vi "Autonomous Independent.vi"   [LabVIEW 2012]
doc: "This VI is called when autonomous begins, and will automatically be terminated when autonomous ends. You can carry out timed or sensor driven robot movement independently without needing to return to the caller."
uses:
  <vilib>/Rock Robotics/WPI/CAN/Jaguar/SubVIs/WPI_CANJaguar_ControlMode.ctl
  <vilib>/Rock Robotics/WPI/CAN/Jaguar/SubVIs/WPI_CANJaguar_PositionReference.ctl
  <vilib>/Rock Robotics/WPI/CAN/Jaguar/SubVIs/WPI_CANJaguar_SpeedReference.ctl
  Robot Global Data.vi
  <vilib>/Rock Robotics/WPI/Solenoid/Deprecated/WPI_SolenoidSetBool.vi
  <vilib>/Rock Robotics/WPI/Joystick/WPI_JoystickGetSetRefNum.vi
types:
  T1 = typedef "WPI_JoystickDevRef.ctl" = cluster{"Device":T2}
  T2 = typedef "WPI_JoystickDeviceEnum.ctl" = enum16{"USB 1", "USB 2", "USB 3", "USB 4", "Kinect 1", "Kinect 2"}
  T3 = cluster{"axis 1 (x)":dbl, "axis 2 (y)":dbl, "axis 3 (throttle)":dbl, "axis 4":dbl, "axis 5":dbl, "axis 6":dbl}
  T4 = typedef "WPI_MotorControlDeviceRef.ctl" = cluster{"DeviceStatus":errorcluster, "Type":enum16{"PWM", "CAN"}, "PWM":cluster{"Digital Module":T5, "PWM Channel":T6, "DeadBand":T7}, "CAN":cluster{"Device Number":u8, "Control Mode":T8, "Semaphore":T9, "Max Vout":dbl}, "Invert":bool, "TransformRef":T10, "InvTransformRef":T10}
  T5 = typedef "FPGA_TypedefDigitalModule.ctl" = enum16{"Digital Module 1", "Digital Module 2"}
  T6 = typedef "FPGA_DIOPWMChannel.ctl" = enum8{"PWM 1", "PWM 2", "PWM 3", "PWM 4", "PWM 5", "PWM 6", "PWM 7", "PWM 8", "PWM 9", "PWM 10", "Invalid"}
  T7 = typedef "WPI_PWMDeadband.ctl" = cluster{"Name":string, "maxPositivePwm":i32, "minPositivePwm":i32, "centerPwm":i32, "maxNegativePwm":i32, "minNegativePwm":i32, "angularRange":u16}
  T8 = typedef "WPI_CANJaguar_ControlMode.ctl" = enum8{"Percent VBus", "Current", "Speed", "Position", "Voltage"}
  T9 = typedef "Semaphore RefNum" = refnum<k1>
  T10 = typedef "WPI_PWMTransform_ConPane.ctl" = refnum<vi>
  T11 = typedef "WPI_SolenoidDevRef.ctl" = cluster{"DevStatus":errorcluster, "Solenoid Module":T12, "Forward Solenoid Channel":T13, "Reverse Solenoid Channel":T13}
  T12 = typedef "FPGA_TypedefSolenoidModule.ctl" = enum16{"Solenoid Module 1", "Solenoid Module 2"}
  T13 = typedef "WPI_SolenoidChannel.ctl" = enum8{"Solenoid 1", "Solenoid 2", "Solenoid 3", "Solenoid 4", "Solenoid 5", "Solenoid 6", "Solenoid 7", "Solenoid 8", "Invalid"}
  T14 = typedef "WPI_CANJaguar_PositionReference.ctl" = u8
  T15 = typedef "WPI_CANJaguar_SpeedReference.ctl" = u8
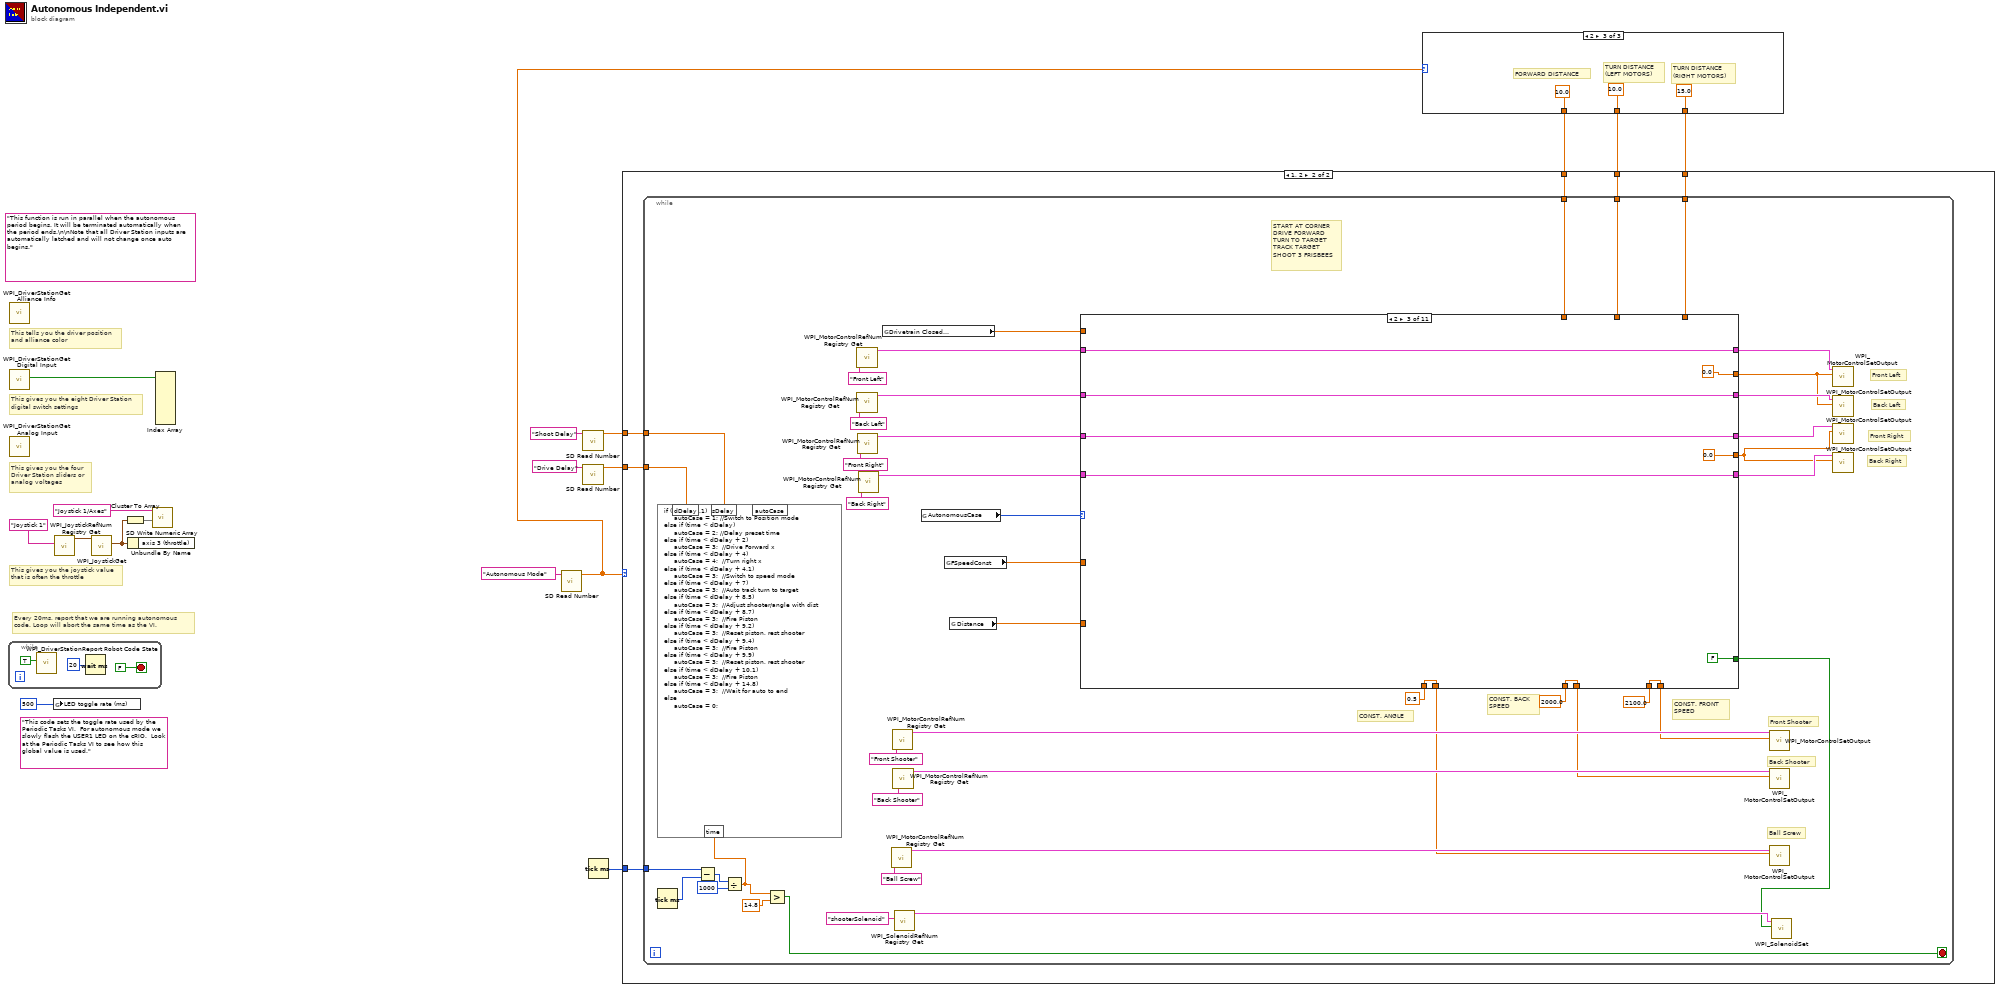
[diagram p0: block diagram]
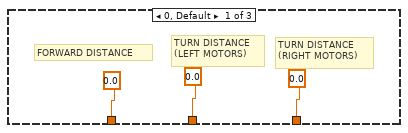
[diagram p2: hidden frame]
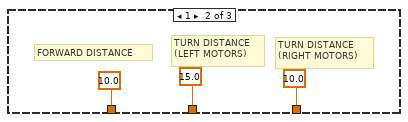
[diagram p3: hidden frame]
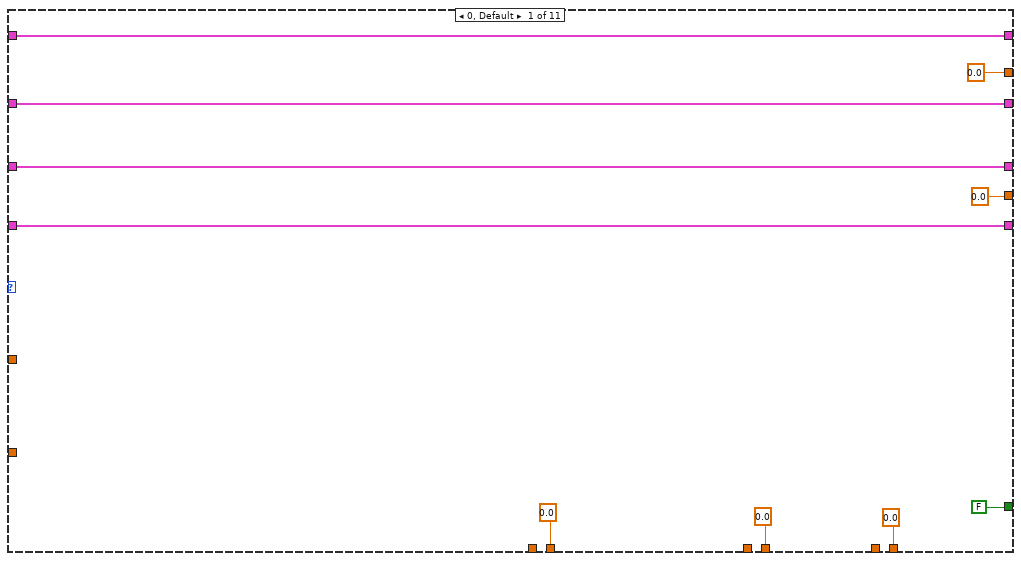
[diagram p5: hidden frame]
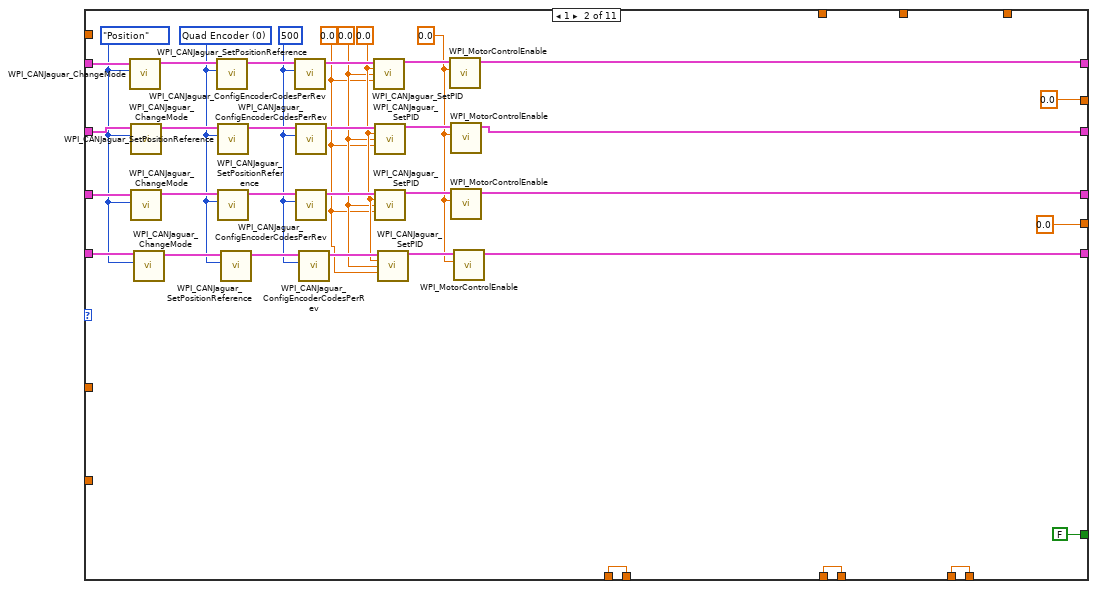
[diagram p6: hidden frame]
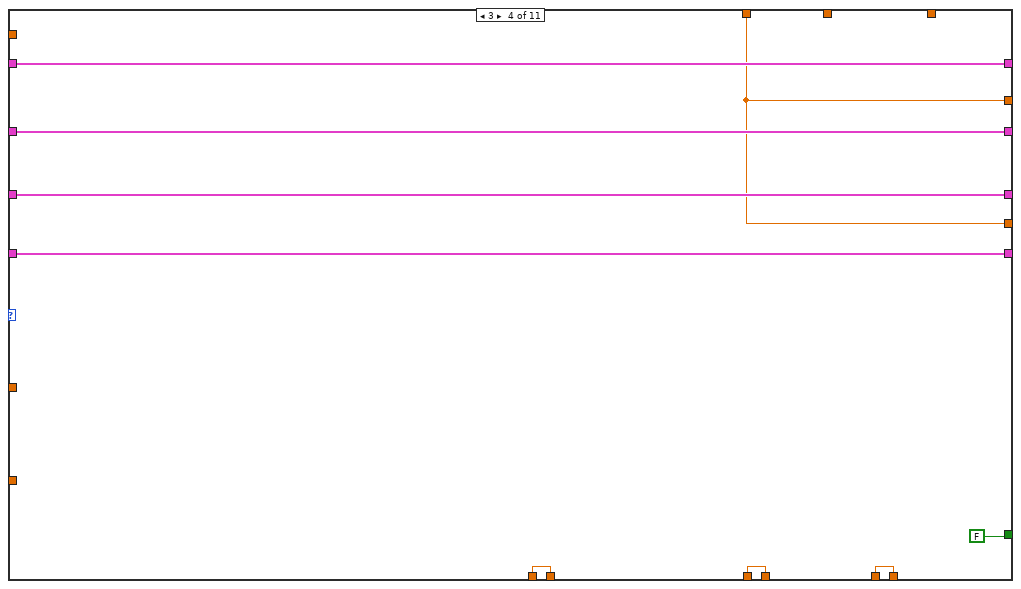
[diagram p7: hidden frame]
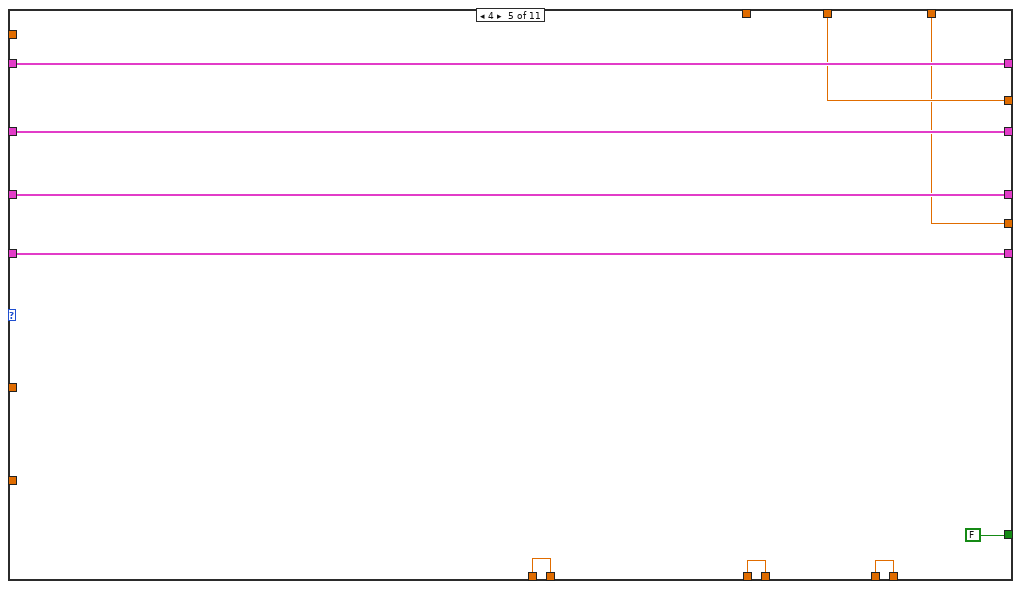
[diagram p8: hidden frame]
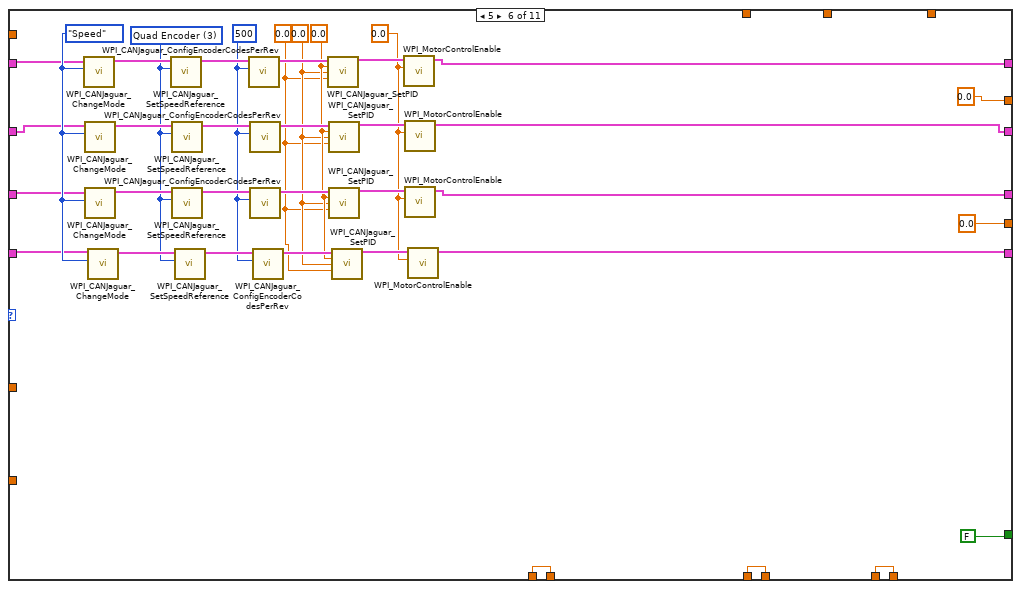
[diagram p9: hidden frame]
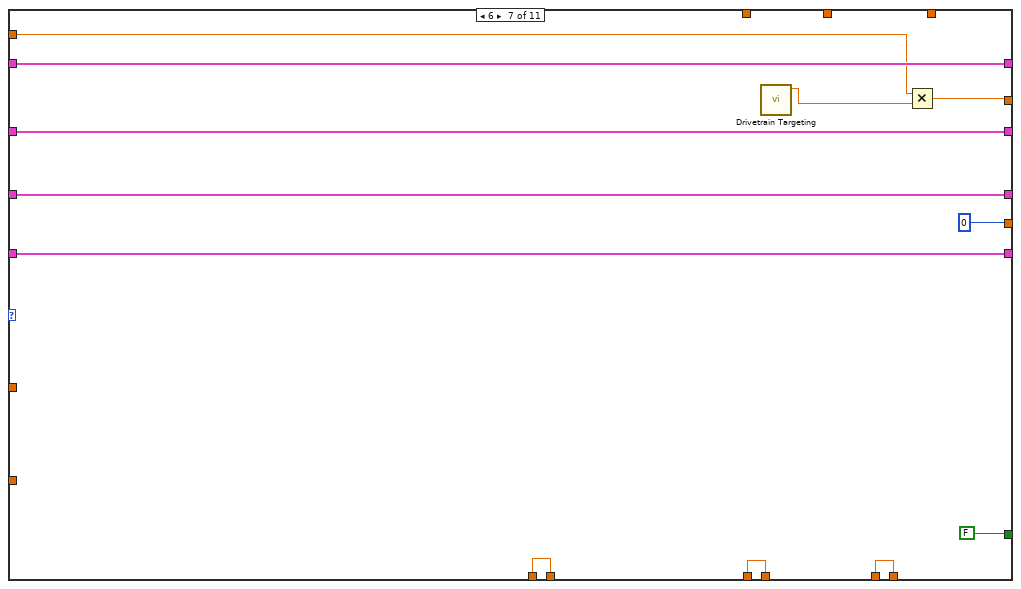
[diagram p10: hidden frame]
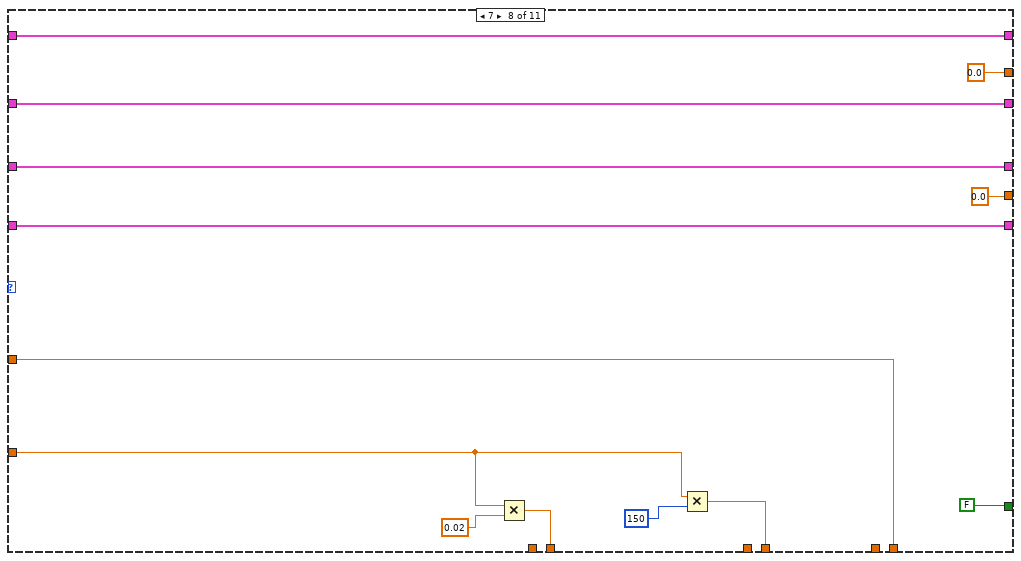
[diagram p11: hidden frame]
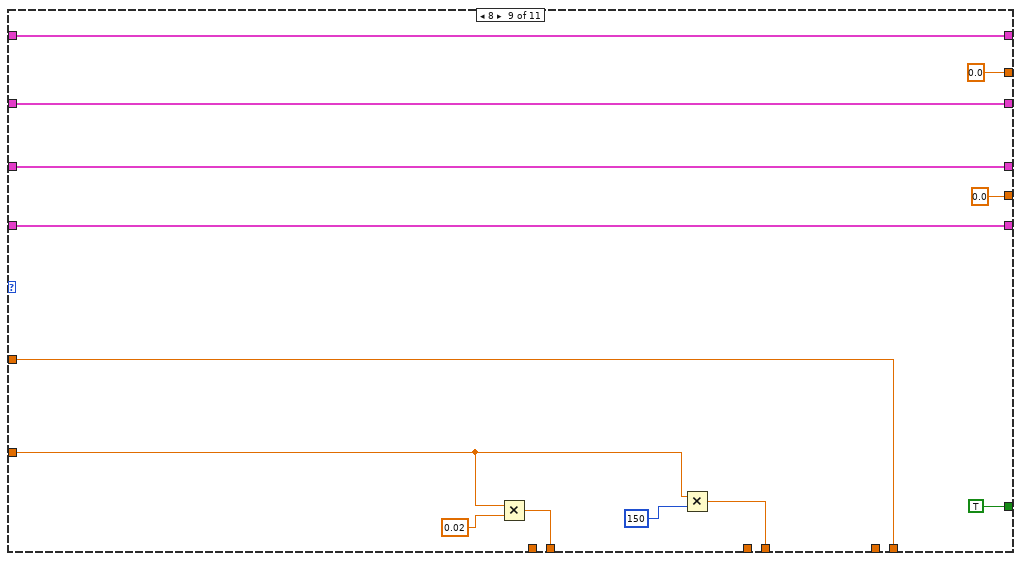
[diagram p12: hidden frame]
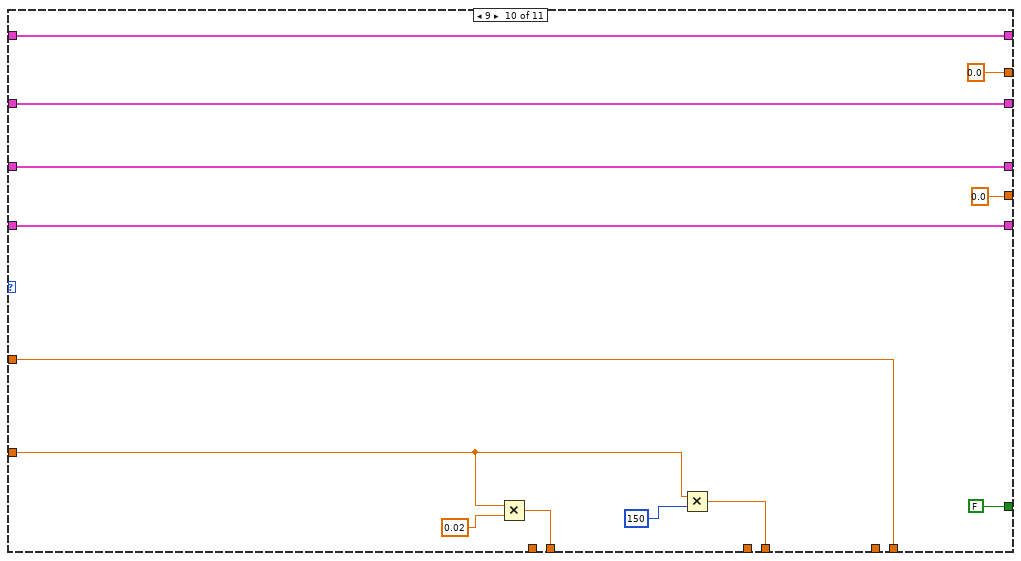
[diagram p13: hidden frame]
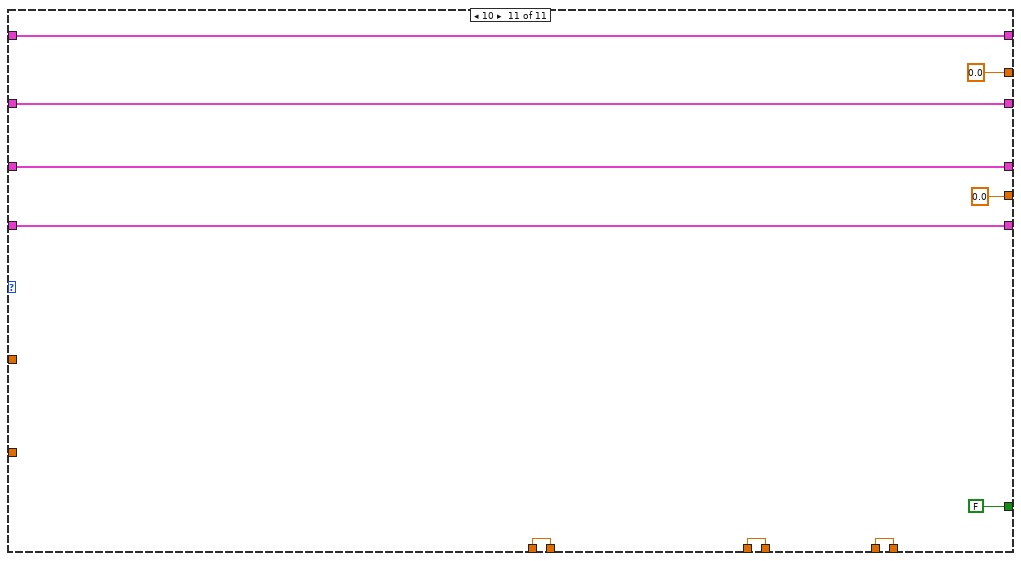
[diagram p14: hidden frame]
diagram:
  (unwired) "This code sets the toggle rate used by the Periodic Tasks VI.  For autonomous mode we slowly flash the USER1 LED on the cRIO.  Look at the Periodic Tasks VI to see how this global value is used."
  (unwired) "This function is run in parallel when the autonomous period begins. It will be terminated automatically when the period ends.\n\nNote that all Driver Station inputs are automatically latched and will not change once auto begins."
  # "Every 20ms, report that we are running autonomous\ncode. Loop will abort the same time as the VI."
  # "This gives you the joystick value\nthat is often the throttle"
  # "This tells you the driver position\nand alliance color"
  # "This gives you the eight Driver Station\ndigital switch settings"
  # "This gives you the four\nDriver Station sliders or\nanalog voltages"
  n1 = while {
    stop <- FALSE stop-if-true
    n2 = call <vilib>:"WPI_DriverStationReport Robot Code State.vi"("Autonomous"=TRUE) -> ()  [unwired: 10 in, 1 out]
    n3 = Wait (ms)(milliseconds to wait=u32 20) -> ()  [unwired: 1 out]
  }
  n4 = call <vilib>:"WPI_DriverStationGet Alliance Info.vi"() -> ()  [unwired: 12 out]
  n5 = call <vilib>:"WPI_DriverStationGet Digital Input.vi"() -> ("Driver Station Digital Input (1-8)"=w17:bool[])  [unwired: 11 out]
  n6 = call <vilib>:"WPI_DriverStationGet Analog Input.vi"() -> ()  [unwired: 12 out]
  n7 = global write "Robot Global Data.vi" "LED toggle rate (ms)"(u32 500 ("LED ms toggle rate")) -> ()
  n8 = call <vilib>:"WPI_JoystickRefNum Registry Get.vi"("refnum name"="Joystick 1") -> ("JoystickDevRef"=w15:T1)  [unwired: 1 in, 9 out]
  n9 = call <vilib>:"WPI_JoystickGet.vi"("JoystickDevRef"=w15) -> ("Axes"=w12:T3)  [unwired: 1 in, 5 out]
  n10 = Cluster To Array(cluster=w12) -> (array=w13:dbl[])
  n11 = Unbundle By Name(w12) -> ()  [unwired: 1 out]
  n12 = call <vilib>:"SD Write Numeric Array.vi"("Numeric Array"=w13, "Name"="Joystick 1/Axes") -> ()  [unwired: 8 in, 2 out]
  n13 = Index Array(array=w17) -> ()  [unwired: 8 in, 8 out]
  n14 = call <vilib>:"SD Read Number.vi"("Name"="Autonomous Mode") -> ("Numeric"=w1:dbl)  [unwired: 8 in, 2 out]
  n15 = call <vilib>:"SD Read Number.vi"("Name"="Shoot Delay") -> ("Numeric"=w5:dbl)  [unwired: 8 in, 2 out]
  n16 = call <vilib>:"SD Read Number.vi"("Name"="Drive Delay") -> ("Numeric"=w6:dbl)  [unwired: 8 in, 2 out]
  n17 = Tick Count (ms)() -> (millisecond timer value=w9:u32)
  n18 = case shown="2" w1 {
    tunnel: [0.0 ("Output") 10.0 ("Output") 10.0 ("Output")] -> w4
    tunnel: [0.0 ("Output") 15.0 ("Output") 10.0 ("Output")] -> w3
    tunnel: [0.0 ("Output") 10.0 ("Output") 15.0 ("Output")] -> w2
    frame 0, Default {
      # "TURN DISTANCE\n(RIGHT MOTORS)"
      # "TURN DISTANCE\n(LEFT MOTORS)"
      # "FORWARD DISTANCE"
    }
    frame 1 {
      # "TURN DISTANCE\n(RIGHT MOTORS)"
      # "TURN DISTANCE\n(LEFT MOTORS)"
      # "FORWARD DISTANCE"
    }
    frame 2 {
      # "TURN DISTANCE\n(RIGHT MOTORS)"
      # "TURN DISTANCE\n(LEFT MOTORS)"
      # "FORWARD DISTANCE"
    }
  }
  n19 = case shown="1, 2" w1 {
    tunnel: w9 -> [_ w35]
    tunnel: w6 -> [_ w34]
    tunnel: w5 -> [_ w33]
    tunnel: w4 -> [_ w32]
    tunnel: w3 -> [_ w31]
    tunnel: w2 -> [_ w30]
    frame 0, Default {
    }
    frame 1, 2 {
      n20 = while {
        tunnel: w35 -> [w44]
        tunnel: w34 -> [w41]
        tunnel: w33 -> [w40]
        tunnel: w32 -> [w38]
        tunnel: w31 -> [w37]
        tunnel: w30 -> [w36]
        stop <- w42 stop-if-true
        # "START AT CORNER\nDRIVE FORWARD\nTURN TO TARGET\nTRACK TARGET\nSHOOT 3 FRISBEES"
        # "CONST. BACK\nSPEED"
        # "CONST. FRONT\nSPEED"
        # "CONST. ANGLE"
        # "Back Right"
        # "Front Right"
        # "Back Left"
        # "Front Left"
        # "Front Shooter"
        # "Back Shooter"
        # "Ball Screw"
        n21 = Tick Count (ms)() -> (millisecond timer value=w43:u32)
        n22 = Subtract(x=w44, y=w43) -> (x-y=w47:u32)
        n23 = Divide(x=w47, y=u32 1000) -> (x/y=w39:dbl)
        n24 = formula code="if (time < 0.1)\n     autoCase = 1; //Switch to Position mode\nelse if (time < dDelay)\n     autoCase = 2; //Delay preset time\nelse if (time < dDelay + 2)\n     autoCase = 3;  //Drive Forward x\nelse if (time < dDelay + 4)\n     autoCase = 4;  //Turn right x\nelse if (time < dDelay + 4.1)\n     autoCase = 3;  //Switch to speed mode\nelse if (time < dDelay + 7)\n     autoCase = 3;  //Auto track turn to target\nelse if (time < dDelay + 8.5)\n     autoCase = 3;  //Adjust shooter/angle with dist\nelse if (time < dDelay + 8.7)\n     autoCase = 3;  //Fire Piston\nelse if (time < dDelay + 9.2)\n     autoCase = 3;  //Reset piston, rest shooter\nelse if (time < dDelay + 9.4)\n     autoCase = 3;  //Fire Piston\nelse if (time < dDelay + 9.9)\n     autoCase = 3;  //Reset piston, rest shooter\nelse if (time < dDelay + 10.1)\n     autoCase = 3;  //Fire Piston\nelse if (time < dDelay + 14.8)\n     autoCase = 3;  //Wait for auto to end\nelse\n     autoCase = 0;"("time"=w39, "dDelay"=w41, "sDelay"=w40) -> ()  [unwired: 1 out]
        n25 = Greater?(x=w39, y=14.8) -> (0:w42:bool)
        n26 = call <vilib>:"WPI_MotorControlRefNum Registry Get.vi"("refnum name"="Front Left") -> ("MotorControlDevRef"=w71:T4)  [unwired: 9 in, 1 out]
        n27 = call <vilib>:"WPI_MotorControlRefNum Registry Get.vi"("refnum name"="Back Left") -> ("MotorControlDevRef"=w69:T4)  [unwired: 9 in, 1 out]
        n28 = call <vilib>:"WPI_MotorControlRefNum Registry Get.vi"("refnum name"="Front Right") -> ("MotorControlDevRef"=w67:T4)  [unwired: 9 in, 1 out]
        n29 = call <vilib>:"WPI_MotorControlRefNum Registry Get.vi"("refnum name"="Back Right") -> ("MotorControlDevRef"=w65:T4)  [unwired: 9 in, 1 out]
        n30 = global read "Robot Global Data.vi" "Drivetrain Closed\nLoop Max"() -> (w53:dbl)
        n31 = call <vilib>:"WPI_MotorControlRefNum Registry Get.vi"("refnum name"="Ball Screw") -> ("MotorControlDevRef"=w60:T4)  [unwired: 9 in, 1 out]
        n32 = call <vilib>:"WPI_MotorControlRefNum Registry Get.vi"("refnum name"="Front Shooter") -> ("MotorControlDevRef"=w62:T4)  [unwired: 9 in, 1 out]
        n33 = call <vilib>:"WPI_MotorControlRefNum Registry Get.vi"("refnum name"="Back Shooter") -> ("MotorControlDevRef"=w61:T4)  [unwired: 9 in, 1 out]
        n34 = call <vilib>:"WPI_SolenoidRefNum Registry Get.vi"("refnum name"="shooterSolenoid") -> ("SolenoidDevRef"=w49:T11)  [unwired: 9 in, 1 out]
        n35 = global read "Robot Global Data.vi" "AutonomousCase"() -> (w80:i8)
        n36 = global read "Robot Global Data.vi" "FSpeedConst"() -> (w51:dbl)
        n37 = global read "Robot Global Data.vi" "Distance"() -> (w52:dbl)
        n38 = case shown="2" w80 {
          tunnel: [w88 w100 w137 w146 w156 w162 w205 w216 w229 w242 w252] -> w72
          tunnel: w71 -> [w88 w127 w137 w146 w156 w163 w205 w216 w229 w242 w252]
          tunnel: [w87 w99 w136 w145 w155 w161 w204 w215 w228 w241 w251] -> w70
          tunnel: w69 -> [w87 w108 w136 w145 w155 w164 w204 w215 w228 w241 w251]
          tunnel: [w86 w98 w135 w144 w154 w160 w203 w214 w227 w240 w250] -> w68
          tunnel: w67 -> [w86 w109 w135 w144 w154 w165 w203 w214 w227 w240 w250]
          tunnel: [w85 w97 w134 w143 w153 w159 w202 w213 w226 w239 w249] -> w66
          tunnel: w65 -> [w85 w110 w134 w143 w153 w166 w202 w213 w226 w239 w249]
          tunnel: [0.0 ("P") 0.0 ("P") 0.0 ("Output") w142 w152 0.0 ("Output") w198 0.0 ("P") 0.0 ("P") 0.0 ("P") 0.0 ("P")] -> w64
          tunnel: [0.0 ("P") 0.0 ("P") 0.0 ("Output") w142 w151 0.0 ("Output") 0 0.0 ("P") 0.0 ("P") 0.0 ("P") 0.0 ("P")] -> w63
          tunnel: [0.0 ("P") w92 w129 w139 w148 w189 w199 w210 w223 w236 w245] -> w59
          tunnel: [0.0 ("P") w93 w130 w140 w149 w190 w200 w207 w220 w233 w246] -> w58
          tunnel: [0.0 ("P") w94 w131 w141 w150 w191 w201 w211 w224 w237 w247] -> w57
          tunnel: w38 -> [_ _ _ w142 _ _ _ _ _ _ _]
          tunnel: w37 -> [_ _ _ _ w152 _ _ _ _ _ _]
          tunnel: w36 -> [_ _ _ _ w151 _ _ _ _ _ _]
          tunnel: 0.5 ("P") -> [_ w94 w131 w141 w150 w191 w201 _ _ _ w247]
          tunnel: 2000.0 ("P") -> [_ w93 w130 w140 w149 w190 w200 _ _ _ w246]
          tunnel: 2100.0 ("P") -> [_ w92 w129 w139 w148 w189 w199 _ _ _ w245]
          tunnel: w53 -> [_ _ _ _ _ _ w197 _ _ _ _]
          tunnel: w52 -> [_ _ _ _ _ _ _ w208 w221 w234 _]
          tunnel: w51 -> [_ _ _ _ _ _ _ w210 w223 w236 _]
          tunnel: [FALSE FALSE FALSE FALSE FALSE FALSE FALSE FALSE TRUE FALSE FALSE] -> w48
          frame 0, Default {
          }
          frame 1 {
            w101 = 0.0 ("P")
            w102 = 0.0 ("P")
            w103 = 0.0 ("P")
            w104 = 0.0 ("P")
            w105 = u16 500 ("Encoder Codes Per Rev")
            w106 = T14 0 items=["Quad Encoder"=0, "Potentiometer"=1, "None"=255] ("Position Reference")
            w107 = WPI_CANJaguar_ControlMode."Position" ("Control Mode")
            n39 = call <vilib>:"WPI_CANJaguar_ChangeMode.vi"("Control Mode"=w107, "CAN Jaguar Ref"=w127) -> ("CAN Jaguar Ref Out"=w126:T4)  [unwired: 8 in, 1 out]
            n40 = call <vilib>:"WPI_CANJaguar_ChangeMode.vi"("Control Mode"=w107, "CAN Jaguar Ref"=w108) -> ("CAN Jaguar Ref Out"=w122:T4)  [unwired: 8 in, 1 out]
            n41 = call <vilib>:"WPI_CANJaguar_ChangeMode.vi"("Control Mode"=w107, "CAN Jaguar Ref"=w109) -> ("CAN Jaguar Ref Out"=w118:T4)  [unwired: 8 in, 1 out]
            n42 = call <vilib>:"WPI_CANJaguar_ChangeMode.vi"("Control Mode"=w107, "CAN Jaguar Ref"=w110) -> ("CAN Jaguar Ref Out"=w114:T4)  [unwired: 8 in, 1 out]
            n43 = call <vilib>:"WPI_CANJaguar_SetPositionReference.vi"("Position Reference"=w106, "CAN Jaguar Ref"=w126) -> ("CAN Jaguar Ref Out"=w125:T4)  [unwired: 8 in, 1 out]
            n44 = call <vilib>:"WPI_CANJaguar_SetPositionReference.vi"("Position Reference"=w106, "CAN Jaguar Ref"=w122) -> ("CAN Jaguar Ref Out"=w121:T4)  [unwired: 8 in, 1 out]
            n45 = call <vilib>:"WPI_CANJaguar_SetPositionReference.vi"("Position Reference"=w106, "CAN Jaguar Ref"=w118) -> ("CAN Jaguar Ref Out"=w117:T4)  [unwired: 8 in, 1 out]
            n46 = call <vilib>:"WPI_CANJaguar_SetPositionReference.vi"("Position Reference"=w106, "CAN Jaguar Ref"=w114) -> ("CAN Jaguar Ref Out"=w113:T4)  [unwired: 8 in, 1 out]
            n47 = call <vilib>:"WPI_CANJaguar_ConfigEncoderCodesPerRev.vi"("Encoder Codes Per Rev"=w105, "CAN Jaguar Ref"=w125) -> ("CAN Jaguar Ref Out"=w124:T4)  [unwired: 8 in, 1 out]
            n48 = call <vilib>:"WPI_CANJaguar_ConfigEncoderCodesPerRev.vi"("Encoder Codes Per Rev"=w105, "CAN Jaguar Ref"=w121) -> ("CAN Jaguar Ref Out"=w120:T4)  [unwired: 8 in, 1 out]
            n49 = call <vilib>:"WPI_CANJaguar_ConfigEncoderCodesPerRev.vi"("Encoder Codes Per Rev"=w105, "CAN Jaguar Ref"=w117) -> ("CAN Jaguar Ref Out"=w116:T4)  [unwired: 8 in, 1 out]
            n50 = call <vilib>:"WPI_CANJaguar_ConfigEncoderCodesPerRev.vi"("Encoder Codes Per Rev"=w105, "CAN Jaguar Ref"=w113) -> ("CAN Jaguar Ref Out"=w112:T4)  [unwired: 8 in, 1 out]
            n51 = call <vilib>:"WPI_CANJaguar_SetPID.vi"("CAN Jaguar Ref"=w124, "P"=w104, "I"=w103, "D"=w102) -> ("CAN Jaguar Ref Out"=w123:T4)  [unwired: 10 in, 1 out]
            n52 = call <vilib>:"WPI_CANJaguar_SetPID.vi"("CAN Jaguar Ref"=w120, "P"=w104, "I"=w103, "D"=w102) -> ("CAN Jaguar Ref Out"=w119:T4)  [unwired: 10 in, 1 out]
            n53 = call <vilib>:"WPI_CANJaguar_SetPID.vi"("CAN Jaguar Ref"=w116, "P"=w104, "I"=w103, "D"=w102) -> ("CAN Jaguar Ref Out"=w115:T4)  [unwired: 10 in, 1 out]
            n54 = call <vilib>:"WPI_CANJaguar_SetPID.vi"("CAN Jaguar Ref"=w112, "P"=w104, "I"=w103, "D"=w102) -> ("CAN Jaguar Ref Out"=w111:T4)  [unwired: 10 in, 1 out]
            n55 = call <vilib>:"WPI_MotorControlEnable.vi"("Encoder Initial Position"=w101, "CAN Jaguar Ref"=w123) -> ("CAN Jaguar Ref Out"=w100:T4)  [unwired: 8 in, 1 out]
            n56 = call <vilib>:"WPI_MotorControlEnable.vi"("Encoder Initial Position"=w101, "CAN Jaguar Ref"=w119) -> ("CAN Jaguar Ref Out"=w99:T4)  [unwired: 8 in, 1 out]
            n57 = call <vilib>:"WPI_MotorControlEnable.vi"("Encoder Initial Position"=w101, "CAN Jaguar Ref"=w115) -> ("CAN Jaguar Ref Out"=w98:T4)  [unwired: 8 in, 1 out]
            n58 = call <vilib>:"WPI_MotorControlEnable.vi"("Encoder Initial Position"=w101, "CAN Jaguar Ref"=w111) -> ("CAN Jaguar Ref Out"=w97:T4)  [unwired: 8 in, 1 out]
          }
          frame 2 {
          }
          frame 3 {
          }
          frame 4 {
          }
          frame 5 {
            w158 = T15 3 items=["Encoder"=0, "Inv Encoder"=2, "Quad Encoder"=3, "None"=255] ("Speed Reference")
            w167 = 0.0 ("P")
            w168 = 0.0 ("P")
            w169 = 0.0 ("P")
            w170 = 0.0 ("P")
            w171 = u16 500 ("Encoder Codes Per Rev")
            w172 = WPI_CANJaguar_ControlMode."Speed" ("Control Mode")
            n59 = call <vilib>:"WPI_CANJaguar_ChangeMode.vi"("Control Mode"=w172, "CAN Jaguar Ref"=w163) -> ("CAN Jaguar Ref Out"=w188:T4)  [unwired: 8 in, 1 out]
            n60 = call <vilib>:"WPI_CANJaguar_ChangeMode.vi"("Control Mode"=w172, "CAN Jaguar Ref"=w164) -> ("CAN Jaguar Ref Out"=w184:T4)  [unwired: 8 in, 1 out]
            n61 = call <vilib>:"WPI_CANJaguar_ChangeMode.vi"("Control Mode"=w172, "CAN Jaguar Ref"=w165) -> ("CAN Jaguar Ref Out"=w180:T4)  [unwired: 8 in, 1 out]
            n62 = call <vilib>:"WPI_CANJaguar_ChangeMode.vi"("Control Mode"=w172, "CAN Jaguar Ref"=w166) -> ("CAN Jaguar Ref Out"=w176:T4)  [unwired: 8 in, 1 out]
            n63 = call <vilib>:"WPI_CANJaguar_SetSpeedReference.vi"("Speed Reference"=w158, "CAN Jaguar Ref"=w188) -> ("CAN Jaguar Ref Out"=w187:T4)  [unwired: 8 in, 1 out]
            n64 = call <vilib>:"WPI_CANJaguar_SetSpeedReference.vi"("Speed Reference"=w158, "CAN Jaguar Ref"=w184) -> ("CAN Jaguar Ref Out"=w183:T4)  [unwired: 8 in, 1 out]
            n65 = call <vilib>:"WPI_CANJaguar_SetSpeedReference.vi"("Speed Reference"=w158, "CAN Jaguar Ref"=w180) -> ("CAN Jaguar Ref Out"=w179:T4)  [unwired: 8 in, 1 out]
            n66 = call <vilib>:"WPI_CANJaguar_SetSpeedReference.vi"("Speed Reference"=w158, "CAN Jaguar Ref"=w176) -> ("CAN Jaguar Ref Out"=w175:T4)  [unwired: 8 in, 1 out]
            n67 = call <vilib>:"WPI_CANJaguar_ConfigEncoderCodesPerRev.vi"("Encoder Codes Per Rev"=w171, "CAN Jaguar Ref"=w187) -> ("CAN Jaguar Ref Out"=w186:T4)  [unwired: 8 in, 1 out]
            n68 = call <vilib>:"WPI_CANJaguar_ConfigEncoderCodesPerRev.vi"("Encoder Codes Per Rev"=w171, "CAN Jaguar Ref"=w183) -> ("CAN Jaguar Ref Out"=w182:T4)  [unwired: 8 in, 1 out]
            n69 = call <vilib>:"WPI_CANJaguar_ConfigEncoderCodesPerRev.vi"("Encoder Codes Per Rev"=w171, "CAN Jaguar Ref"=w179) -> ("CAN Jaguar Ref Out"=w178:T4)  [unwired: 8 in, 1 out]
            n70 = call <vilib>:"WPI_CANJaguar_ConfigEncoderCodesPerRev.vi"("Encoder Codes Per Rev"=w171, "CAN Jaguar Ref"=w175) -> ("CAN Jaguar Ref Out"=w174:T4)  [unwired: 8 in, 1 out]
            n71 = call <vilib>:"WPI_CANJaguar_SetPID.vi"("CAN Jaguar Ref"=w186, "P"=w170, "I"=w169, "D"=w168) -> ("CAN Jaguar Ref Out"=w185:T4)  [unwired: 10 in, 1 out]
            n72 = call <vilib>:"WPI_CANJaguar_SetPID.vi"("CAN Jaguar Ref"=w182, "P"=w170, "I"=w169, "D"=w168) -> ("CAN Jaguar Ref Out"=w181:T4)  [unwired: 10 in, 1 out]
            n73 = call <vilib>:"WPI_CANJaguar_SetPID.vi"("CAN Jaguar Ref"=w178, "P"=w170, "I"=w169, "D"=w168) -> ("CAN Jaguar Ref Out"=w177:T4)  [unwired: 10 in, 1 out]
            n74 = call <vilib>:"WPI_CANJaguar_SetPID.vi"("CAN Jaguar Ref"=w174, "P"=w170, "I"=w169, "D"=w168) -> ("CAN Jaguar Ref Out"=w173:T4)  [unwired: 10 in, 1 out]
            n75 = call <vilib>:"WPI_MotorControlEnable.vi"("Encoder Initial Position"=w167, "CAN Jaguar Ref"=w185) -> ("CAN Jaguar Ref Out"=w162:T4)  [unwired: 8 in, 1 out]
            n76 = call <vilib>:"WPI_MotorControlEnable.vi"("Encoder Initial Position"=w167, "CAN Jaguar Ref"=w181) -> ("CAN Jaguar Ref Out"=w161:T4)  [unwired: 8 in, 1 out]
            n77 = call <vilib>:"WPI_MotorControlEnable.vi"("Encoder Initial Position"=w167, "CAN Jaguar Ref"=w177) -> ("CAN Jaguar Ref Out"=w160:T4)  [unwired: 8 in, 1 out]
            n78 = call <vilib>:"WPI_MotorControlEnable.vi"("Encoder Initial Position"=w167, "CAN Jaguar Ref"=w173) -> ("CAN Jaguar Ref Out"=w159:T4)  [unwired: 8 in, 1 out]
          }
          frame 6 {
            n79 = call "Drivetrain Targeting.vi"() -> ("X Axis Out"=w196:dbl)  [unwired: 11 in]
            n80 = Multiply(x=w197, y=w196) -> (x*y=w198:dbl)
          }
          frame 7 {
            n81 = Multiply(x=w208, y=0.02) -> (x*y=w211:dbl)
            n82 = Multiply(x=w208, y=150) -> (x*y=w207:dbl)
          }
          frame 8 {
            n83 = Multiply(x=w221, y=0.02) -> (x*y=w224:dbl)
            n84 = Multiply(x=w221, y=150) -> (x*y=w220:dbl)
          }
          frame 9 {
            n85 = Multiply(x=w234, y=0.02) -> (x*y=w237:dbl)
            n86 = Multiply(x=w234, y=150) -> (x*y=w233:dbl)
          }
          frame 10 {
          }
        }
        n87 = call <vilib>:"WPI_MotorControlSetOutput.vi"("Output"=w59, "MotorControlDevRef"=w62) -> ()  [unwired: 7 in, 3 out]
        n88 = call <vilib>:"WPI_MotorControlSetOutput.vi"("Output"=w58, "MotorControlDevRef"=w61) -> ()  [unwired: 7 in, 3 out]
        n89 = call <vilib>:"WPI_MotorControlSetOutput.vi"("Output"=w57, "MotorControlDevRef"=w60) -> ()  [unwired: 7 in, 3 out]
        n90 = call-poly <vilib>:"WPI_SolenoidSet.vi"("Value"=w48, "SolenoidDevRef"=w49) -> ()  [unwired: 8 in, 2 out]
        n91 = call <vilib>:"WPI_MotorControlSetOutput.vi"("Output"=w64, "MotorControlDevRef"=w72) -> ()  [unwired: 7 in, 3 out]
        n92 = call <vilib>:"WPI_MotorControlSetOutput.vi"("Output"=w64, "MotorControlDevRef"=w70) -> ()  [unwired: 7 in, 3 out]
        n93 = call <vilib>:"WPI_MotorControlSetOutput.vi"("Output"=w63, "MotorControlDevRef"=w68) -> ()  [unwired: 7 in, 3 out]
        n94 = call <vilib>:"WPI_MotorControlSetOutput.vi"("Output"=w63, "MotorControlDevRef"=w66) -> ()  [unwired: 7 in, 3 out]
      }
    }
  }
